vi "Initialize Plot Property Page.vi"(6 "Plot Area Ref":refnum<vi>, 8 "error in (no error)":errorcluster, 9 "2D Error Bar Array In":T3, 11 "Plot Property Array In":T1) -> (0 "error out":errorcluster, 1 "2D Error Bar Array Out":T3, 3 "Plot Property Array Out":T1)   [LabVIEW 2017, in "2D Error Bar.lvclass"]
uses:
  <vilib>/Math Plots/2D Math Plots/2D Error Bar/2D Error Bar/2D Error Bar.lvclass
  <vilib>/Math Plots/2D Math Plots/2D Error Bar/2D Error Bar/Typedef/2D Error Bar Property Array.ctl
  <vilib>/Math Plots/2D Math Plots/2D Error Bar/2D Error Bar/Typedef/2D Error Bar Property.ctl
  <vilib>/Math Plots/2D Math Plots/2D Plot/2D Plot/Typedef/Plot Property Array.ctl
  <vilib>/Math Plots/2D Math Plots/2D Plot/2D Plot/Typedef/Plot Property.ctl
  <vilib>/Math Plots/2D Math Plots/2D Plot/2D Plot/2D Plot.lvclass
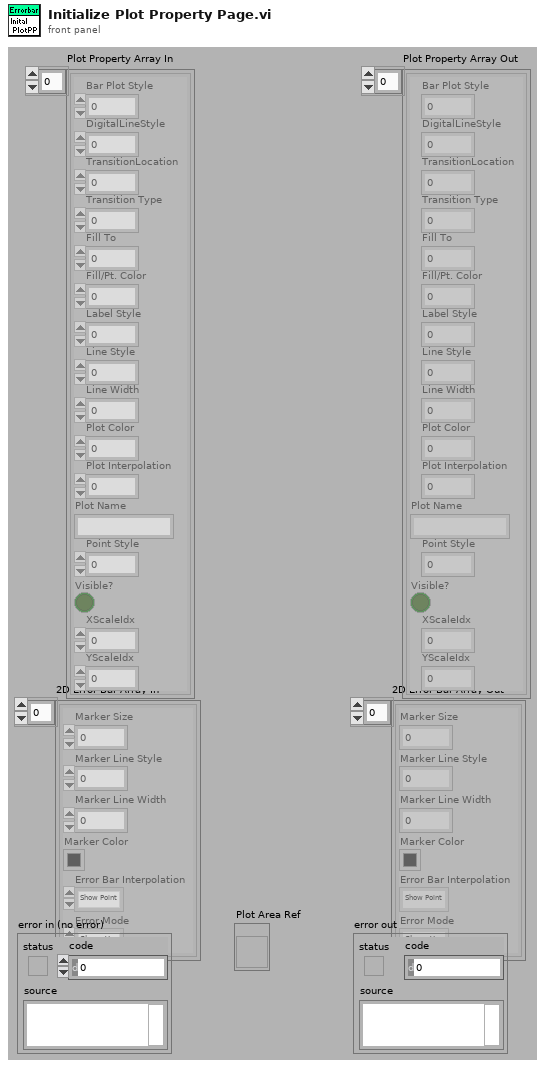
[diagram p1: front panel]
types:
  T1 = typedef "2D Plot.lvclass/Plot Property Array.ctl" = T2[]
  T2 = typedef "2D Plot.lvclass/Plot Property.ctl" = cluster{"Bar Plot Style":u8, "DigitalLineStyle":u8, "TransitionLocation":u8, "Transition Type":u8, "Fill To":i16, "Fill/Pt. Color":u32, "Label Style":u8, "Line Style":u8, "Line Width":u8, "Plot Color":u32, "Plot Interpolation":u8, "Plot Name":string, "Point Style":u8, "Visible?":bool, "XScaleIdx":u32, "YScaleIdx":u32}
  T3 = typedef "2D Error Bar.lvclass/2D Error Bar Property Array.ctl" = T4[]
  T4 = typedef "2D Error Bar.lvclass/2D Error Bar Property.ctl" = cluster{"Marker Size":dbl, "Marker Line Style":u8, "Marker Line Width":u8, "Marker Color":u32, "Error Bar Interpolation":enum16{"Show Point", "Show Line", "Show Bar"}, "Error Mode":enum16{"Show Y Error", "Show X Error", "Show Both Error"}}
  T5 = enum16{"Show Y Error", "Show X Error", "Show Both Error"}
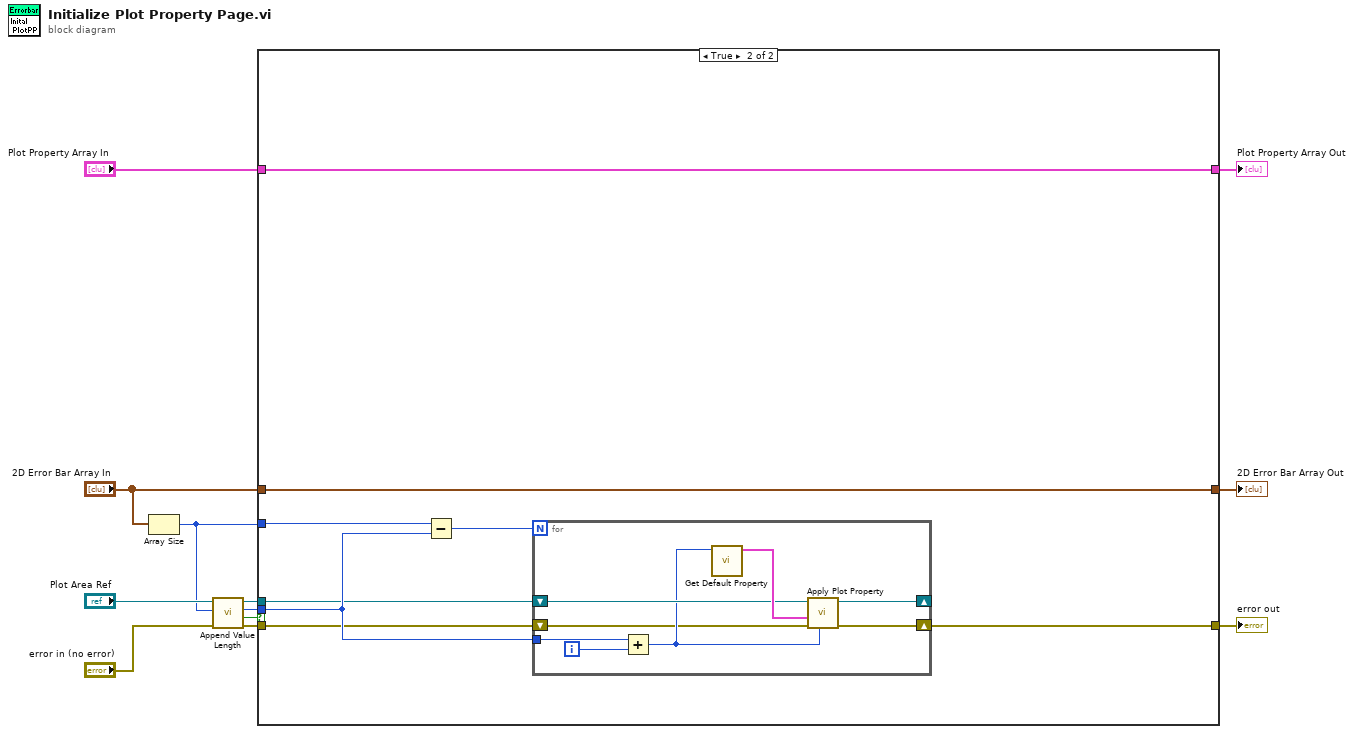
[diagram p0: block diagram]
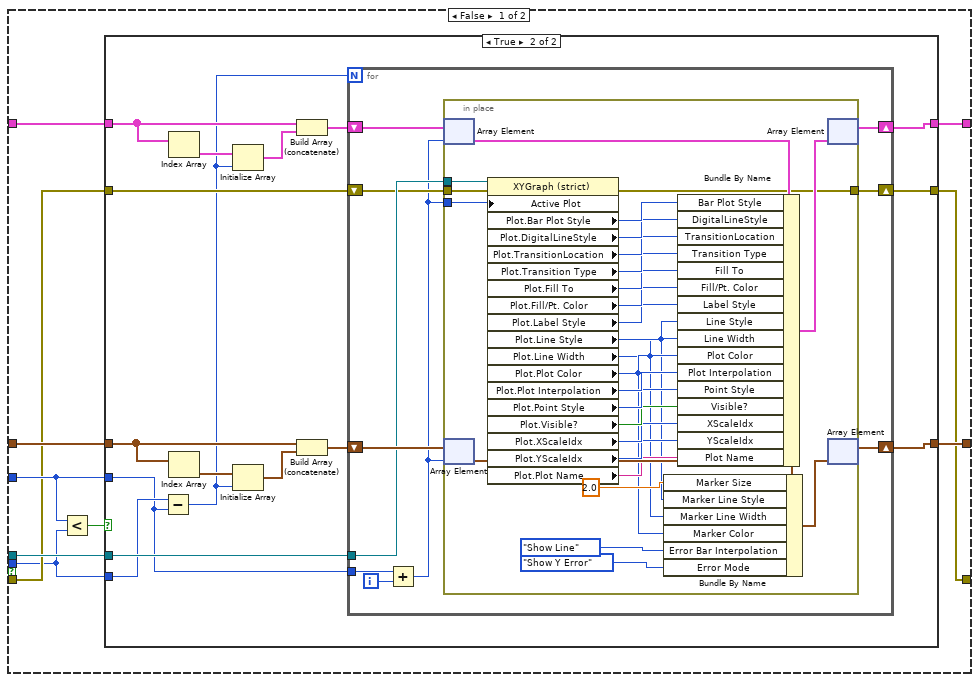
[diagram p2: hidden frame]
diagram:
  n1 = Array Size(array="2D Error Bar Array In") -> (size(s)=w2:i32)
  n2 = call <vilib>:"Append Value Length.vi"("error in (no error)"="error in (no error)", "Expect Value Length"=w2, "Plot Area Ref In"="Plot Area Ref") -> ("error out"=w4:errorcluster, "Append Value?"=w1:bool, "Actual Value Length"=w3:i32, "Plot Area Ref Out"=w5:refnum<vi>)  [unwired: 1 in, 4 out]
  n3 = case shown="True" w1 {
    tunnel: "Plot Property Array In" -> [w21 w86]
    tunnel: [w22 w86] -> w11
    tunnel: "2D Error Bar Array In" -> [w19 w85]
    tunnel: [w20 w85] -> w12
    tunnel: w5 -> [w17 w80]
    tunnel: w2 -> [w16 w84]
    tunnel: w4 -> [w15 w79]
    tunnel: [w14 w83] -> w8
    tunnel: w3 -> [w13 w82]
    frame False {
      n4 = Less?(x=w16, y=w13) -> (x < y?=w18:bool)
      n5 = case shown="True" w18 {
        tunnel: [w25 w34] -> w22
        tunnel: w21 -> [w25 w37]
        tunnel: [w24 w33] -> w20
        tunnel: w19 -> [w24 w29]
        tunnel: w17 -> [_ w41]
        tunnel: w16 -> [_ w35]
        tunnel: w13 -> [_ w40]
        tunnel: w15 -> [w23 w28]
        tunnel: [w23 w27] -> w14
        frame False {
        }
        frame True {
          n6 = Subtract(x=w40, y=w35) -> (x-y=w26:i32)
          n7 = Index Array(array=w37) -> (element=w39:T2)  [unwired: 1 in]
          n8 = Index Array(array=w29) -> (element=w31:T4)  [unwired: 1 in]
          n9 = Initialize Array(w39, w26) -> (w38:T2[])
          n10 = Initialize Array(w31, w26) -> (w32:T4[])
          n11 = Build Array (concatenate)(w37, w38) -> (w36:T1)
          n12 = Build Array (concatenate)(w29, w32) -> (w30:T3)
          n13 = for {
            N: w26 -> [_]
            tunnel: w41 -> [w45]
            tunnel: w35 -> [w51]
            shift-right: [w48] -> w34
            shift-left: w36 -> [w49]
            shift-right: [w47] -> w33
            shift-left: w30 -> [w50]
            shift-right: [w43] -> w27
            shift-left: w28 -> [w44]
            i -> [w46]
            n14 = Add(x=w51, y=w46) -> (x+y=w42:i32)
            n15 = in-place {
              in-place-border: w45 -> [w73]
              in-place-border: w42 -> [w72]
              in-place-border: w44 -> [w59]
              in-place-border: [w58] -> w43
              n16 = in-place-array #1(w49, w42) -> (w78:T2)
              n17 = in-place-array #2(w50, w42) -> (w76:T4)
              n18 = property class="XYGraph (strict)"(reference=w73, error in=w59, "Active Plot"=w72) -> (error out=w58:errorcluster, "Plot.Bar Plot Style"=w71:u8, "Plot.DigitalLineStyle"=w70:u8, "Plot.TransitionLocation"=w69:u8, "Plot.Transition Type"=w68:u8, "Plot.Fill To"=w67:i16, "Plot.Fill/Pt. Color"=w66:u32, "Plot.Label Style"=w65:u8, "Plot.Line Style"=w54:u8, "Plot.Line Width"=w53:u8, "Plot.Plot Color"=w55:u32, "Plot.Plot Interpolation"=w64:u8, "Plot.Point Style"=w63:u8, "Plot.Visible?"=w62:bool, "Plot.XScaleIdx"=w61:u32, "Plot.YScaleIdx"=w60:u32, "Plot.Plot Name"=w57:string)  [unwired: 1 out]
              n19 = Bundle By Name(cluster=w76, "Marker Size"=2.0 ("Arrow Size"), "Marker Line Style"=w54, "Marker Line Width"=w53, "Marker Color"=w55, "Error Bar Interpolation"=enum16{"Show Point", "Show Line", "Show Bar"}."Show Line", "Error Mode"=T5."Show Y Error") -> (w75:T4)
              n20 = Bundle By Name(cluster=w78, "Bar Plot Style"=w71, "DigitalLineStyle"=w70, "TransitionLocation"=w69, "Transition Type"=w68, "Fill To"=w67, "Fill/Pt. Color"=w66, "Label Style"=w65, "Line Style"=w54, "Line Width"=w53, "Plot Color"=w55, "Plot Interpolation"=w64, "Point Style"=w63, "Visible?"=w62, "XScaleIdx"=w61, "YScaleIdx"=w60, "Plot Name"=w57) -> (w77:T2)
              n21 = in-place-array #1(w77) -> (w48:T1)  [unwired: 1 out]
              n22 = in-place-array #2(w75) -> (w47:T3)  [unwired: 1 out]
            }
          }
        }
      }
    }
    frame True {
      n23 = Subtract(x=w84, y=w82) -> (x-y=w81:i32)
      n24 = for {
        N: w81 -> [_]
        tunnel: w82 -> [w92]
        shift-right: [w94] -> w83
        shift-left: w79 -> [w87]
        shift-right: [w91] -> _
        shift-left: w80 -> [w89]
        i -> [w93]
        n25 = Add(x=w92, y=w93) -> (x+y=w88:i32)
        n26 = call <vilib>:"Get Default Property.vi"("Index"=w88) -> ("Temporary Property"=w90:T2)  [unwired: 3 in, 7 out]
        n27 = call <vilib>:"Apply Plot Property.vi"("Plot ID"=w88, "error in (no error)"=w87, "Plot Property"=w90, "Polar Area Ref In"=w89) -> ("error out"=w94:errorcluster, "Polar Area Ref Out"=w91:refnum<vi>)  [unwired: 1 in, 5 out]
      }
    }
  }
  "2D Error Bar Array Out" <- w12
  "Plot Property Array Out" <- w11
  "error out" <- w8
